vi "testRunWithAssertionFailure.vi"() -> (0 "error out":errorcluster)   [LabVIEW 2019, in "TestResultTest.lvlib"]
uses:
  TestResultTest.lvlib
  TestResult/TestResult.lvclass
  TestResultTestSupport/TestCaseMock/TestCaseMock.lvclass/TestCaseMock.ctl
  TestResultTestSupport/TestCaseMock/TestCaseMock.lvclass
  C:/Users/de200256/Code/LVUnit/TestCase/TestCase/TestCase.lvclass
  Assertion/Assertion.lvlib
  TestFailure/TestFailure.lvclass
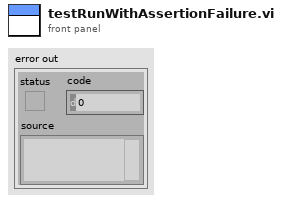
[diagram p1: front panel]
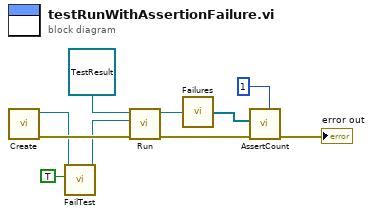
[diagram p0: block diagram]
diagram:
  n1 = call "Create.vi"() -> ("error out"=w9:errorcluster, "TestCaseMock"=w8:refnum<class "TestCaseMock.lvclass">)  [unwired: 10 in]
  n2 = call "FailTest.vi"("Fail Test"=TRUE, "TestCaseMock in"=w8) -> ("TestCaseMock out"=w6:refnum<class "TestCaseMock.lvclass">)  [unwired: 9 in]
  n3 = call-dynamic "Run.vi"("error in (no error)"=w9, "TestCase"=w6, "TestResult in"=refnum<class "TestResult.lvclass"> refnum ("TestResult.lvclass")) -> ("error out"=w10:errorcluster, "TestResult out"=w5:refnum<class "TestResult.lvclass">)  [unwired: 6 in, 1 out]
  n4 = call "Failures.vi"("TestResult In"=w5) -> ("Failures"=w3:refnum<class "TestFailure.lvclass">[])
  n5 = call "AssertCount.vi"("Expected"=1, "error in (no error)"=w10, "Haystack"=w3) -> ("error out"=→"error out":errorcluster)  [unwired: 8 in]
